vi "Get Routing Channel Configuration.vi"(8 "error in (no error)":errorcluster, 11 "Channel Ref in":T1 format="%.0x") -> (0 "error out":errorcluster, 1 "State and Connections List":T2, 2 "Channel Name":string, 3 "Channel Ref out":T1 format="%.0x", 4 "Initial State":string, 6 "Description":string)   [LabVIEW 2017, in "Routing and Faulting Scripting.lvlib"]
uses:
  Routing and Faulting Scripting.lvlib
  <vilib>/NI Veristand/Custom Device API/Custom Device Item Ref.ctl
  Shared/Channel States.ctl
  Shared/Routing State.ctl
  Shared/Connection.ctl
  <vilib>/NI VeriStand/Custom Device API/Custom Device API.lvlib
  Shared/Routing and Faulting Shared.lvlib
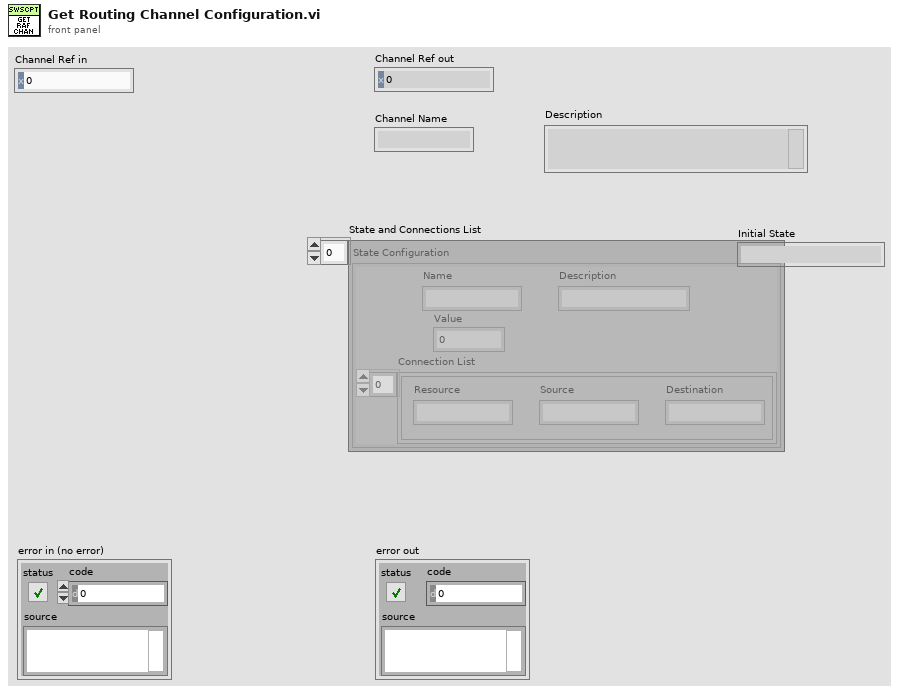
[diagram p1: front panel]
types:
  T1 = typedef "Custom Device API.lvlib/Custom Device Item Ref.ctl" = u64
  T2 = typedef "Routing and Faulting Shared.lvlib/Channel States.ctl" = T3[]
  T3 = typedef "Routing and Faulting Shared.lvlib/Routing State.ctl" = cluster{"Name":string, "Description":string, "Value":i32, "Connection List":T4[]}
  T4 = typedef "Routing and Faulting Shared.lvlib/Connection.ctl" = cluster{"Resource":string, "Source":string, "Destination":string}
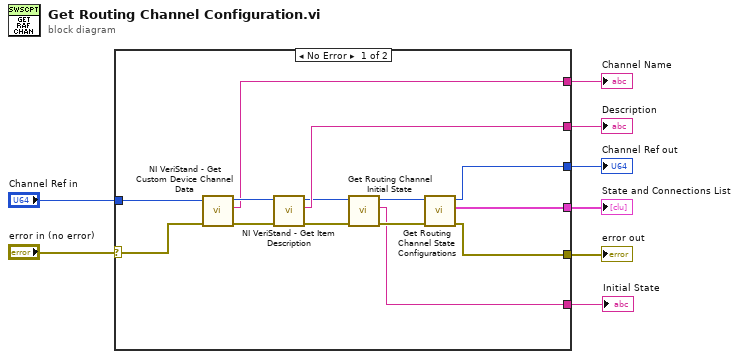
[diagram p0: block diagram]
diagram:
  n1 = case shown="No Error" "error in (no error)" {
    selector: "error in (no error)" -> [w22 w23]
    tunnel: [w20 w23] -> w8
    tunnel: "Channel Ref in" -> [w19 _]
    tunnel: [w15 _] -> w4
    tunnel: [w21 _] -> w5
    tunnel: [w18 _] -> w3
    tunnel: [w14 _] -> w2
    tunnel: [w9 _] -> w1
    frame No Error {
      n2 = call <vilib>:"NI VeriStand - Get Custom Device Channel Data.vi"("error in (no error)"=w22, "Channel Ref in"=w19) -> ("error out"=w16:errorcluster, "Channel Name"=w15:string, "Channel Ref out"=w17:T1)  [unwired: 4 in, 3 out]
      n3 = call <vilib>:"NI VeriStand - Get Item Description.vi"("error in (no error)"=w16, "Item Ref in"=w17) -> ("error out"=w11:errorcluster, "Description"=w14:string, "Item Ref out"=w13:T1)  [unwired: 6 in, 1 out]
      n4 = call "Get Routing Channel Initial State.vi"("error in (no error)"=w11, "Channel Ref in"=w13) -> ("error out"=w10:errorcluster, "Initial State"=w9:string, "Channel Ref out"=w12:T1)  [unwired: 7 in]
      n5 = call "Get Routing Channel State Configurations.vi"("error in (no error)"=w10, "Channel Ref in"=w12) -> ("error out"=w20:errorcluster, "State Configurations"=w21:T2, "Channel Ref out"=w18:T1)  [unwired: 7 in]
    }
    frame Error {
    }
  }
  "error out" <- w8
  "Channel Name" <- w4
  "State and Connections List" <- w5
  "Channel Ref out" <- w3
  "Description" <- w2
  "Initial State" <- w1
